vi "Read Behavior.vi"(8 "error in (no error)":errorcluster, 11 "Attribute.StartupBehavior in":refnum<class "Attribute.StartupBehavior.lvclass">) -> (0 "error out":errorcluster, 2 "Behavior":T1, 3 "Attribute.StartupBehavior out":refnum<class "Attribute.StartupBehavior.lvclass">)   [LabVIEW 2019, in "Attribute.StartupBehavior.lvclass"]
doc: "JKI State Machine Objects (SMO) 1.3.0.56\nJKI - JKI\nCopyright (c) 2017, JKI"
uses:
  Attribute.StartupBehavior.lvclass
  ProcessStartupBehavior.ctl
  Attribute.StartupBehavior.lvclass/Attribute.StartupBehavior.ctl
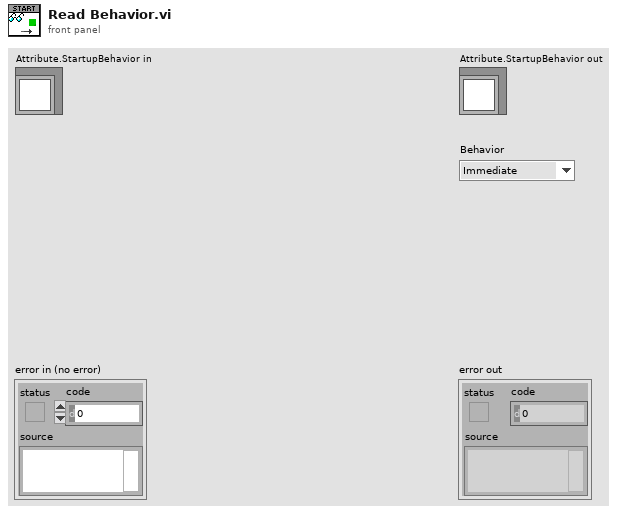
[diagram p1: front panel]
types:
  T1 = typedef "Attribute.StartupBehavior.lvclass/ProcessStartupBehavior.ctl" = enum16{"Immediate", "First Call", "Never"}
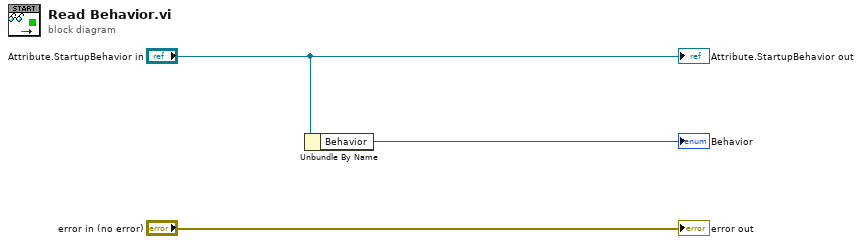
[diagram p0: block diagram]
diagram:
  n1 = Unbundle By Name("Attribute.StartupBehavior in") -> ("Behavior"=→"Behavior":T1)
  "error out" <- "error in (no error)"
  "Attribute.StartupBehavior out" <- "Attribute.StartupBehavior in"
